vi "PSP URL from Variable URL.vi"(8 "error in (no error)":errorcluster, 11 "Shared Variable URL":refnum<k21>) -> (0 "error out":errorcluster, 3 "PSP URL":string)   [LabVIEW 2024]
doc: "Converts a shared variable URL to a PSP URL."
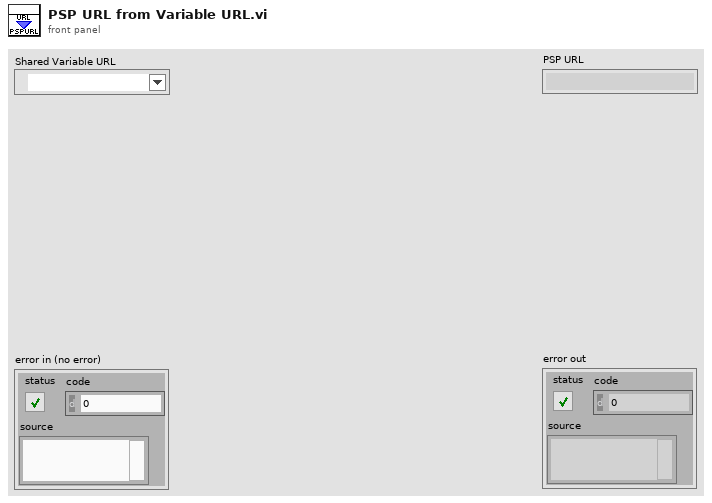
[diagram p1: front panel]
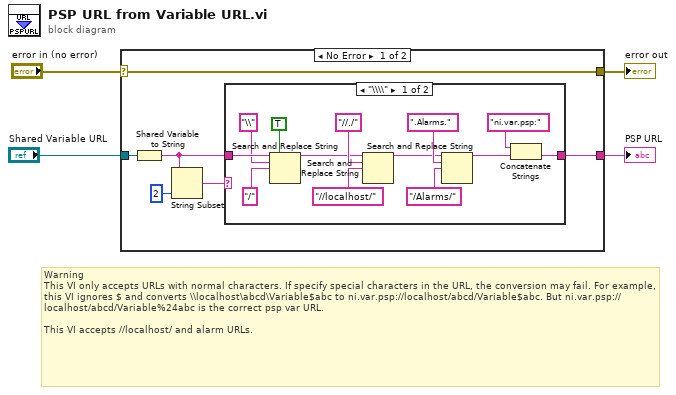
[diagram p0: block diagram]
diagram:
  # "Warning\nThis VI only accepts URLs with normal characters. If specify special characters in the URL, the conversion may fail. For example, this VI ignores $ and converts \\\\localhost\\abcd\\Variable$abc to ni.var.psp://localhost/abcd/Variable$abc. But ni.var.psp://localhost/abcd/Variable%24abc is the correct psp var URL.  \n\nThis VI accepts //localhost/ and alarm URLs."
  n1 = case shown="No Error" "error in (no error)" {
    selector: "error in (no error)" -> [w5 w25]
    tunnel: [w5 w25] -> w3
    tunnel: [w6 _] -> w2
    tunnel: "Shared Variable URL" -> [w7 _]
    frame No Error {
      n2 = Shared Variable to String(1:w7) -> (0:w10:string)
      n3 = String Subset(string=w10, length (rest)=2 ("length (rest)")) -> (substring=w9:string)  [unwired: 1 in]
      n4 = case shown="\"\\\\\\\\\"" w9 {
        tunnel: w10 -> [w23 w24]
        tunnel: [w18 w24] -> w6
        frame "\\\\" {
          n5 = Search and Replace String(replace all?=TRUE ("replace all? (F)"), input string=w23, search string="\\", replace string="/" ("replace string (\"\")")) -> (result string=w15:string)  [unwired: 4 in, 3 out]
          n6 = Search and Replace String(input string=w15, search string="//./", replace string="//localhost/" ("search string")) -> (result string=w11:string)  [unwired: 5 in, 3 out]
          n7 = Search and Replace String(input string=w11, search string=".Alarms.", replace string="/Alarms/" ("search string")) -> (result string=w12:string)  [unwired: 5 in, 3 out]
          n8 = Concatenate Strings("ni.var.psp:" ("search string"), w12) -> (w18:string)
        }
        frame Default {
        }
      }
    }
    frame Error {
    }
  }
  "error out" <- w3
  "PSP URL" <- w2
